vi "Convert TDMS to TDM.vi"(6 "data chunk size":i64=10000000 format="%.0e", 7 "write log file":bool, 8 "error in (no error)":errorcluster, 9 "target file operation (2:create or replace)":T1=enum."create or replace", 10 "target file path (*.tdm)":path, 11 "source file path (*.tdms)":path) -> (0 "error out":errorcluster, 1 "log messages":string, 2 "target file path (*.tdm) out":path, 3 "source file path (*.tdms) out":path)   [LabVIEW 2017]
doc: "LabVIEW no longer supports this VI. Use the Convert to TDM or TDMS VI instead.\n\nConverts the specified file from the .tdms file format to the .tdm file format."
uses:
  <vilib>/Platform/storage/lvStorage.llb/_openFunction.ctl
  <vilib>/Utility/tdmsutil.llb/TDMS2TDMInitializeLog.vi
  <vilib>/Utility/tdmsutil.llb/TDMS2TDMLogIllegalName.vi
  <vilib>/Utility/tdmsutil.llb/TDMS2TDMWriteLogFile.vi
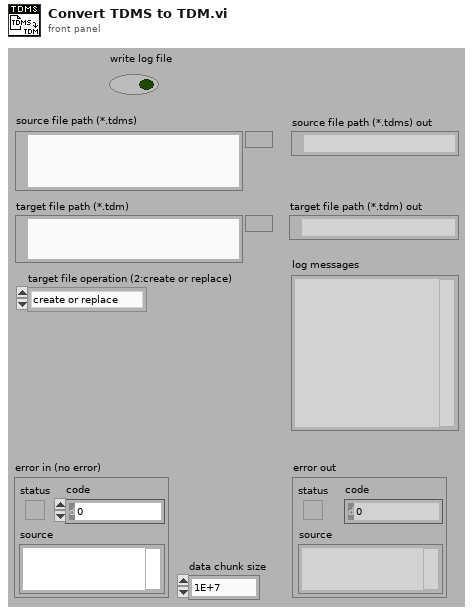
[diagram p1: front panel]
types:
  T1 = typedef "_openFunction.ctl" = enum16{"open", "open or create", "create or replace", "create", "open (read only)"}
  T2 = enum16{"open", "open or create", "create or replace", "create", "open (read-only)"}
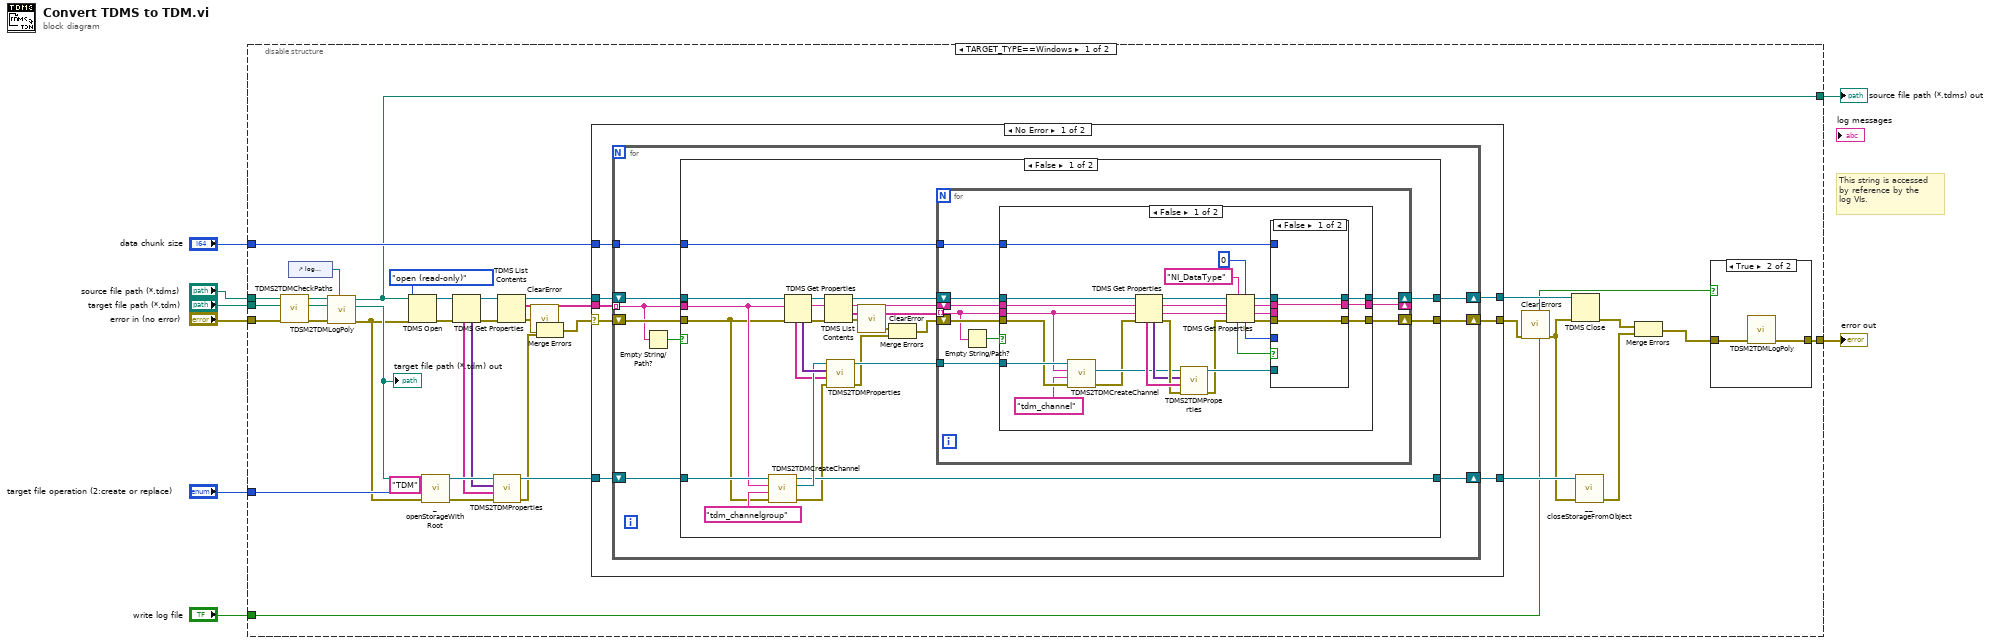
[diagram p0: block diagram]
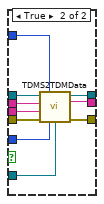
[diagram p3: hidden frame]
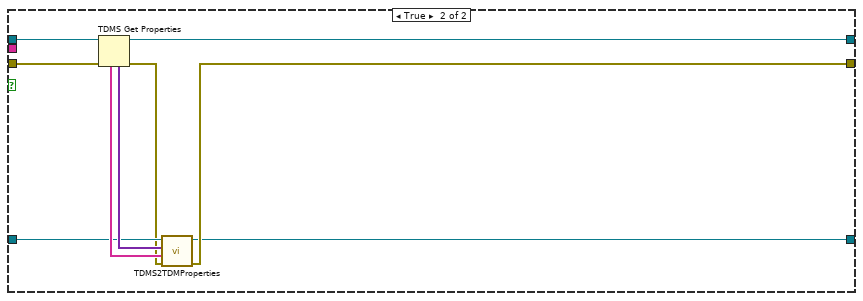
[diagram p5: hidden frame]
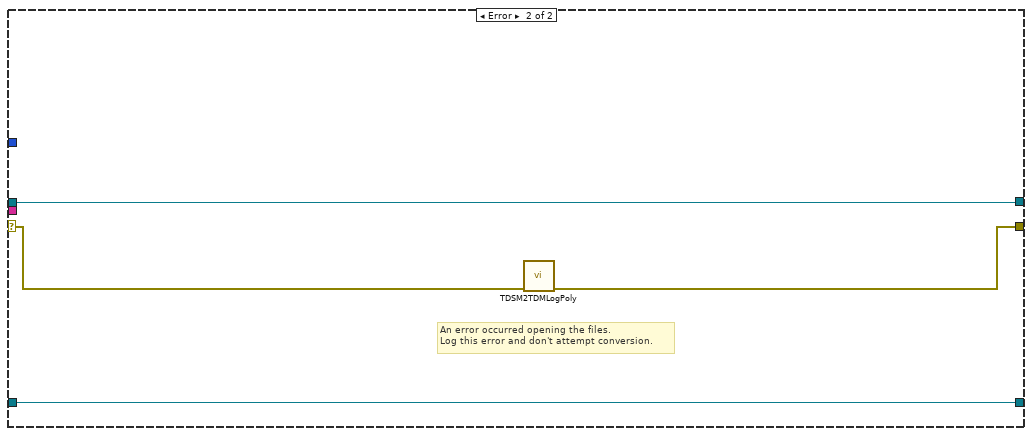
[diagram p6: hidden frame]
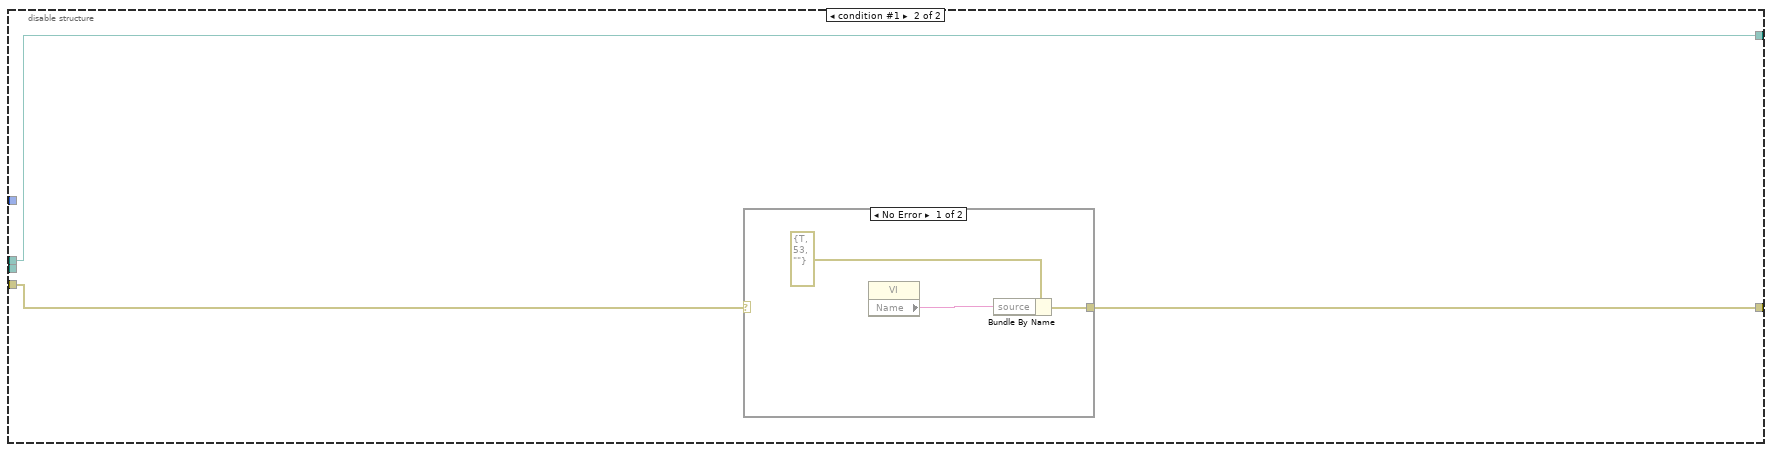
[diagram p7: hidden frame]
diagram:
  # "This string is accessed\nby reference by the\nlog VIs."
  n1 = disable-structure shown="TARGET_TYPE==Windows" {
    disable-tunnel: "target file operation (2:create or replace)" -> [w44 _]
    disable-tunnel: "data chunk size" -> [w40 _]
    disable-tunnel: "source file path (*.tdms)" -> [w37 w158]
    disable-tunnel: "target file path (*.tdm)" -> [w36 _]
    disable-tunnel: "error in (no error)" -> [w35 w159]
    disable-tunnel: "write log file" -> [w34 _]
    disable-tunnel: [w33 w160] -> w2
    disable-tunnel: [w30 w158] -> w1
    frame condition #0 (active) {
      n2 = call <vilib>:"TDMS2TDMCheckPaths.vi"("error in (no error)"=w35, "New TDM Path In"=w36, "TDMS Path In"=w37) -> ("error out"=w26:errorcluster, "New TDM File Out"=w29:path, "TDMS File Out"=w31:path)  [unwired: 6 in]
      n3 = control-ref of="log messages"() -> (w32:refnum<vi>)
      n4 = call-poly <vilib>:"TDSM2TDMLogPoly.vi"("Str Refnum"=w32, "error in (no error)"=w26, "TDM File Path"=w29, "TDMS File Path"=w31) -> ("error out"=w25:errorcluster, "TDM File Path Out"=w28:path, "TDMS File Path Out"=w30:path)  [unwired: 5 in]
      "target file path (*.tdm) out" <- w28
      n5 = TDMS Open(8:w25, 10:T2."open (read-only)" ("TDMS File Operation"), 11:w30) -> (0:w15:errorcluster, 3:w12:refnum<k34>)  [unwired: 4 in]
      n6 = call <vilib>:"_openStorageWithRoot.vi"("error in (no error)"=w25, "Overwrite Options"=w44, "Storage Format"="TDM", "Storage Location"=w28) -> ("error out"=w17:errorcluster, "Data Object"=w19:refnum<k20>)  [unwired: 6 in]
      n7 = TDMS Get Properties(8:w15, 11:w12) -> (0:w14:errorcluster, 3:w13:refnum<k34>, 4:w11:variant[], 6:w10:string[])  [unwired: 4 in, 2 out]
      n8 = call <vilib>:"TDMS2TDMProperties.vi"("error in (no error)"=w17, "property names"=w10, "property values"=w11, "new storage refnum"=w19) -> ("error out"=w16:errorcluster, "new storage refnum out"=w18:refnum<k20>)  [unwired: 6 in]
      n9 = TDMS List Contents(4:w14, 7:w13) -> (0:w9:errorcluster, 2:w20:string[], 3:w45:refnum<k34>)  [unwired: 1 in, 1 out]
      n10 = call <vilib>:"ClearError.vi"("error in (no error)"=w9) -> ("error out"=w39:errorcluster)
      n11 = Merge Errors(w39, w16) -> (w38:errorcluster)
      n12 = case shown="No Error" w38 {
        selector: w38 -> [w51 w155]
        tunnel: w20 -> [w57 _]
        tunnel: w45 -> [w56 w157]
        tunnel: w18 -> [w55 w156]
        tunnel: [w54 w157] -> w43
        tunnel: [w50 w154] -> w27
        tunnel: [w53 w156] -> w42
        tunnel: w40 -> [w52 _]
        frame No Error {
          n13 = for {
            shift-right: [w65] -> w54
            shift-left: w56 -> [w66]
            tunnel: w57 -> [w58] mode=indexing
            shift-right: [w62] -> w53
            shift-left: w55 -> [w63]
            tunnel: w52 -> [w64]
            shift-right: [w61] -> w50
            shift-left: w51 -> [w60]
            n14 = Empty String/Path?(string/path=w58) -> (empty?=w59:bool)
            n15 = case shown="False" w59 {
              tunnel: w66 -> [w90 w151]
              tunnel: [w84 w146] -> w65
              tunnel: w64 -> [w83 _]
              tunnel: w63 -> [w81 w149]
              tunnel: [w79 w145] -> w62
              tunnel: w58 -> [w78 _]
              tunnel: [w77 w147] -> w61
              tunnel: w60 -> [w74 w150]
              frame False {
                n16 = call <vilib>:"TDMS2TDMCreateChannel.vi"("error in (no error)"=w74, "Object type"="tdm_channelgroup", "Name"=w78, "Data Object"=w81) -> ("error out"=w69:errorcluster, "New Storage Refnum"=w80:refnum<k20>, "dup storage refnum"=w79:refnum<k20>)  [unwired: 5 in]
                n17 = TDMS Get Properties(8:w74, 10:w78, 11:w90) -> (0:w73:errorcluster, 2:w88:string, 3:w89:refnum<k34>, 4:w87:variant[], 6:w75:string[])  [unwired: 3 in, 1 out]
                n18 = TDMS List Contents(4:w73, 6:w88, 7:w89) -> (0:w67:errorcluster, 1:w68:string[], 2:w86:string, 3:w85:refnum<k34>)
                n19 = call <vilib>:"TDMS2TDMProperties.vi"("error in (no error)"=w69, "property names"=w75, "property values"=w87, "new storage refnum"=w80) -> ("error out"=w71:errorcluster, "new storage refnum out"=w82:refnum<k20>)  [unwired: 6 in]
                n20 = call <vilib>:"ClearError.vi"("error in (no error)"=w67) -> ("error out"=w72:errorcluster)
                n21 = Merge Errors(w72, w71) -> (w70:errorcluster)
                n22 = for {
                  tunnel: w68 -> [w91] mode=indexing
                  shift-right: [w97] -> _
                  shift-left: w86 -> [w99]
                  shift-right: [w98] -> w84
                  shift-left: w85 -> [w100]
                  tunnel: w83 -> [w96]
                  tunnel: w82 -> [w94]
                  shift-right: [w95] -> w77
                  shift-left: w70 -> [w93]
                  n23 = Empty String/Path?(string/path=w91) -> (empty?=w92:bool)
                  n24 = case shown="False" w92 {
                    tunnel: w100 -> [w126 w144]
                    tunnel: w99 -> [w125 w143]
                    tunnel: [w114 w144] -> w98
                    tunnel: [w113 w143] -> w97
                    tunnel: w96 -> [w112 _]
                    tunnel: [w111 w142] -> w95
                    tunnel: w94 -> [w107 _]
                    tunnel: w93 -> [w106 w142]
                    tunnel: w91 -> [w104 _]
                    frame False {
                      n25 = call <vilib>:"TDMS2TDMCreateChannel.vi"("error in (no error)"=w106, "Object type"="tdm_channel", "Name"=w104, "Data Object"=w107) -> ("error out"=w102:errorcluster, "New Storage Refnum"=w103:refnum<k20>)  [unwired: 5 in, 1 out]
                      n26 = TDMS Get Properties(8:w102, 9:w104, 10:w125, 11:w126) -> (0:w127:errorcluster, 1:w119:string, 2:w120:string, 3:w122:refnum<k34>, 4:w124:variant[], 6:w128:string[])  [unwired: 2 in]
                      n27 = call <vilib>:"TDMS2TDMProperties.vi"("error in (no error)"=w127, "property names"=w128, "property values"=w124, "new storage refnum"=w103) -> ("error out"=w110:errorcluster, "new storage refnum out"=w121:refnum<k20>)  [unwired: 6 in]
                      n28 = TDMS Get Properties(5:0, 7:"NI_DataType" ("property name"), 8:w110, 9:w119, 10:w120, 11:w122) -> (0:w115:errorcluster, 1:w116:string, 2:w117:string, 3:w118:refnum<k34>, 4:w108:i32, 6:w109:bool)
                      n29 = case shown="False" w109 {
                        tunnel: w121 -> [_ w133]
                        tunnel: w118 -> [w131 w141]
                        tunnel: w117 -> [w130 w134]
                        tunnel: w116 -> [_ w140]
                        tunnel: w115 -> [w129 w139]
                        tunnel: [w131 w138] -> w114
                        tunnel: [w130 w132] -> w113
                        tunnel: w112 -> [_ w137]
                        tunnel: [w129 w136] -> w111
                        tunnel: w108 -> [_ w135]
                        frame False {
                        }
                        frame True {
                          n30 = call <vilib>:"TDMS2TDMData.vi"("tdms file in"=w141, "Chunk Size"=w137, "group name"=w134, "channel name"=w140, "error in (no error)"=w139, "Data type"=w135, "storage refnum"=w133) -> ("tdms file out"=w138:refnum<k34>, "group name out"=w132:string, "error out"=w136:errorcluster)  [unwired: 6 in]
                        }
                      }
                    }
                    frame True {
                    }
                  }
                }
              }
              frame True {
                n31 = TDMS Get Properties(8:w150, 11:w151) -> (0:w148:errorcluster, 3:w146:refnum<k34>, 4:w153:variant[], 6:w152:string[])  [unwired: 4 in, 2 out]
                n32 = call <vilib>:"TDMS2TDMProperties.vi"("error in (no error)"=w148, "property names"=w152, "property values"=w153, "new storage refnum"=w149) -> ("error out"=w147:errorcluster, "new storage refnum out"=w145:refnum<k20>)  [unwired: 6 in]
              }
            }
          }
        }
        frame Error {
          # "An error occurred opening the files.\nLog this error and don't attempt conversion."
          n33 = call-poly <vilib>:"TDSM2TDMLogPoly.vi"("error in (no error)"=w155) -> ("error out"=w154:errorcluster)  [unwired: 10 in]
        }
      }
      n34 = call <vilib>:"Clear Errors.vi"("error in (no error)"=w27) -> ("error out"=w24:errorcluster)  [unwired: 5 in, 1 out]
      n35 = TDMS Close(8:w24, 11:w43) -> (0:w23:errorcluster)  [unwired: 1 out]
      n36 = call <vilib>:"__closeStorageFromObject.vi"("error in (no error)"=w24, "storage refnum"=w42) -> ("error out"=w22:errorcluster)  [unwired: 5 in]
      n37 = Merge Errors(w23, w22) -> (w21:errorcluster)
      n38 = case shown="True" w34 {
        tunnel: w21 -> [w47 w49]
        tunnel: [w47 w48] -> w33
        frame False {
        }
        frame True {
          n39 = call-poly <vilib>:"TDSM2TDMLogPoly.vi"("error in (no error)"=w49) -> ("error out"=w48:errorcluster)  [unwired: 10 in]
        }
      }
    }
    frame condition #1 {
      n40 = case shown="No Error" w159 {
        selector: w159 -> [_ w164]
        tunnel: [w162 w164] -> w160
        frame No Error {
          n41 = property class="VI"() -> ("Name"=w161:string)  [unwired: 2 in, 2 out]
          n42 = Bundle By Name(cluster=errorcluster {"status"=TRUE, "code"=53, "source"=""} ("error IO"), "source"=w161) -> (w162:errorcluster)
        }
        frame Error {
        }
      }
    }
  }
  "error out" <- w2
  "source file path (*.tdms) out" <- w1
